vi "Power.vi"(8 "error in":errorcluster, 10 "Power?":bool, 11 "Neph in":refnum<class "Nephelometer.lvclass">) -> (0 "error out":errorcluster, 3 "Neph out":refnum<class "Nephelometer.lvclass">)   [LabVIEW 2014, in "Nephelometer.lvclass"]
uses:
  Nephelometer.lvclass
  Reusable/Session APIs/Serial/Serial Session.lvclass
  Nephelometer.lvclass/Nephelometer.ctl
  Reusable/Session APIs/Text Communication/Text Device Session.lvclass/Text Device Session.ctl
  Accessors/Read Session Handle.vi
  Reusable/Session APIs/Text Communication/Read hSysLog.vi
  <userlib>/_Session Fwk/Session - Root.lvclass
  Reusable/Session Log/System Log.lvclass
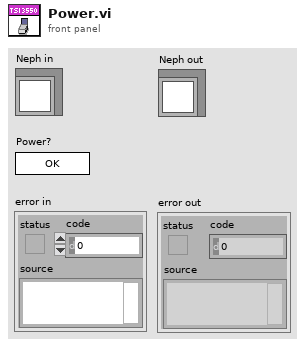
[diagram p1: front panel]
types:
  T1 = typedef "Session - Root.lvclass/Session Handle.ctl" = refnum<data-value>
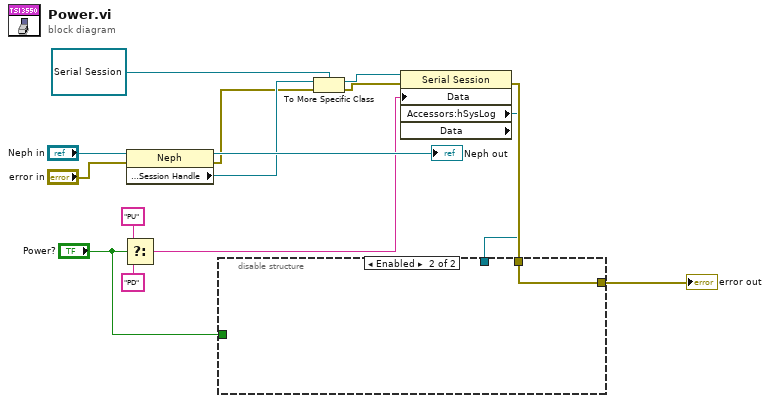
[diagram p0: block diagram]
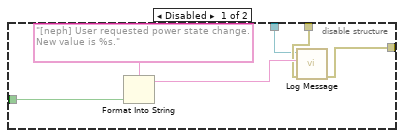
[diagram p2: hidden frame]
diagram:
  n1 = Select(t="PU" ("Write - Asynchronous"), s="Power?", f="PD" ("Write - Asynchronous")) -> (s? t:f=w5:string)
  n2 = property class="Neph"(reference="Neph in", error in="error in") -> (reference out=→"Neph out":refnum<class "Nephelometer.lvclass">, error out=w4:errorcluster, "Accessors:Session Handle"=w6:T1)
  n3 = To More Specific Class(target class=refnum<data-value> refnum ("Session Handle"), reference=w6, error in=w4) -> (specific class reference=w7:refnum<data-value>, error out=w8:errorcluster)
  n4 = property class="Serial Session" props=["Data", "Accessors:hSysLog", "Data"](reference=w7, error in=w8, "Data"=w5) -> (error out=w2:errorcluster, "Accessors:hSysLog"=w1:T1)  [unwired: 2 out]
  n5 = disable-structure shown="Enabled" {
    disable-tunnel: "Power?" -> [w21 _]
    disable-tunnel: [w18 w22] -> w3
    disable-tunnel: w2 -> [w17 w22]
    disable-tunnel: w1 -> [w16 _]
    frame Disabled {
      n6 = Format Into String(format string="[neph] User requested power state change.  New value is %s.", w21) -> (resulting string=w19:string)  [unwired: 2 in, 1 out]
      n7 = call "Log Message.vi"("error in"=w17, "MSG In"=w19, "session in"=w16) -> ("error out"=w18:errorcluster)  [unwired: 7 in, 1 out]
    }
    frame Enabled {
    }
  }
  "error out" <- w3
